vi "Start Streaming Waveforms.vi"(8 "error in (no error)":errorcluster, 10 "WaveformStreamSpecifications":T1[](array[typedef]), 11 "WaveformStreaming in":T2) -> (0 "error out":errorcluster, 3 "WaveformStreaming out":T2)   [LabVIEW 2020, in "NI_VS Waveform Streaming Interface.lvlib"]
doc: "Starts streaming waveform data to the VeriStand Gateway. Use this VI to allow an Event structure to start reading waveform values on the block diagram."
uses:
  <vilib>/NI VeriStand/Execution/WaveformStreaming/NI_VS Waveform Streaming Interface.lvlib
  <vilib>/NI VeriStand/Execution/WaveformStreaming/WaveformStreamingAPI.ctl
  NationalInstruments.VeriStand.ClientAPI
  <vilib>/NI VeriStand/Execution/WaveformStreaming/WaveformStreamSpecification.ctl
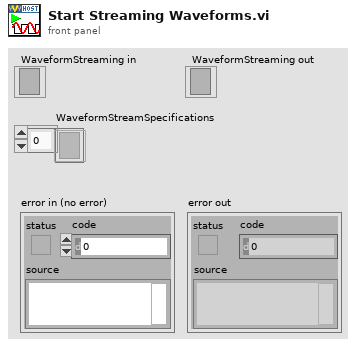
[diagram p1: front panel]
types:
  T1 = typedef "NI_VS Waveform Streaming Interface.lvlib/WaveformStreamSpecification.ctl" = refnum<k24>
  T2 = typedef "NI_VS Waveform Streaming Interface.lvlib/WaveformStreamingAPI.ctl" = refnum<k24>
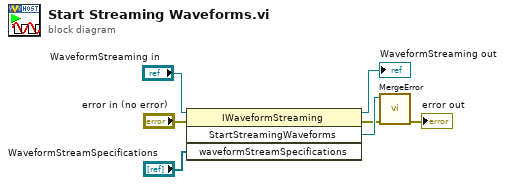
[diagram p0: block diagram]
diagram:
  n1 = invoke class="IWaveformStreaming" method="StartStreamingWaveforms"(reference="WaveformStreaming in", error in="error in (no error)", "waveformStreamSpecifications"="WaveformStreamSpecifications") -> (reference out=→"WaveformStreaming out":T2, error out=w2:errorcluster, "StartStreamingWaveforms"=w3:refnum<k24>)  [unwired: 1 in, 1 out]
  n2 = call <vilib>:"MergeError.vi"("error in (no error)"=w2, "Error"=w3) -> ("error out"=→"error out":errorcluster)  [unwired: 9 in]
